vi "打地鼠.vi"() -> ()   [LabVIEW 2022 SP3]
uses:
  <vilib>/Utility/inputDevices.llb/mouseAcquire.vi
panel:
  out "分数":dbl
  out "goal":bool
  out "行":bool
  out "列":bool
  out "axis info":T1 caption="坐标轴信息"
  out "button info":T2 caption="按钮信息"
  in  "取消按钮":bool
  out "数组":bool[][](array[boolean])
  # "左上角135 160\n右上角535 160\n左下角135 540\n右下角535 540\n\n横着：400/5 = 80\n竖着：380/5 = 76\n\n每个格子，是横80竖76"
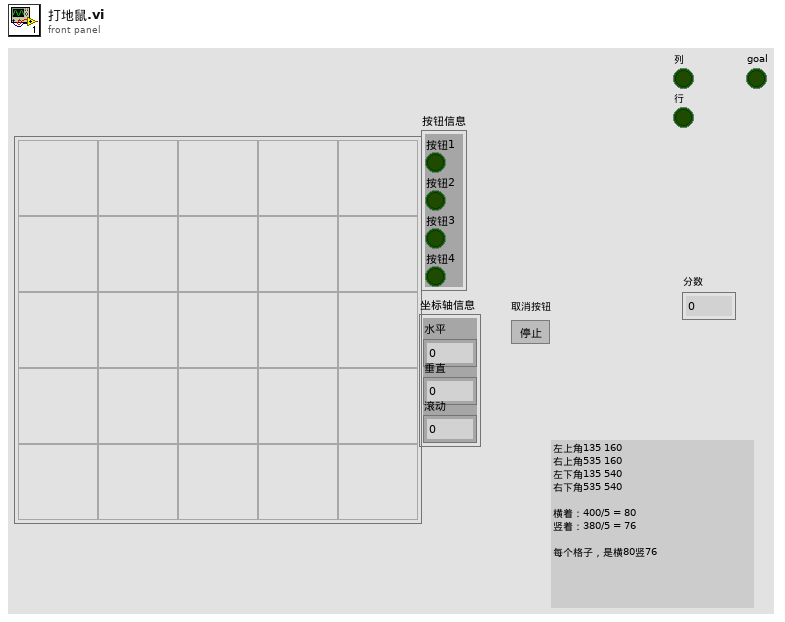
[diagram p1: front panel]
types:
  T1 = cluster{"Horizontal":i32, "Vertical":i32, "Scrolling":i32}
  T2 = cluster{"button 1":bool, "button 2":bool, "button 3":bool, "button 4":bool}
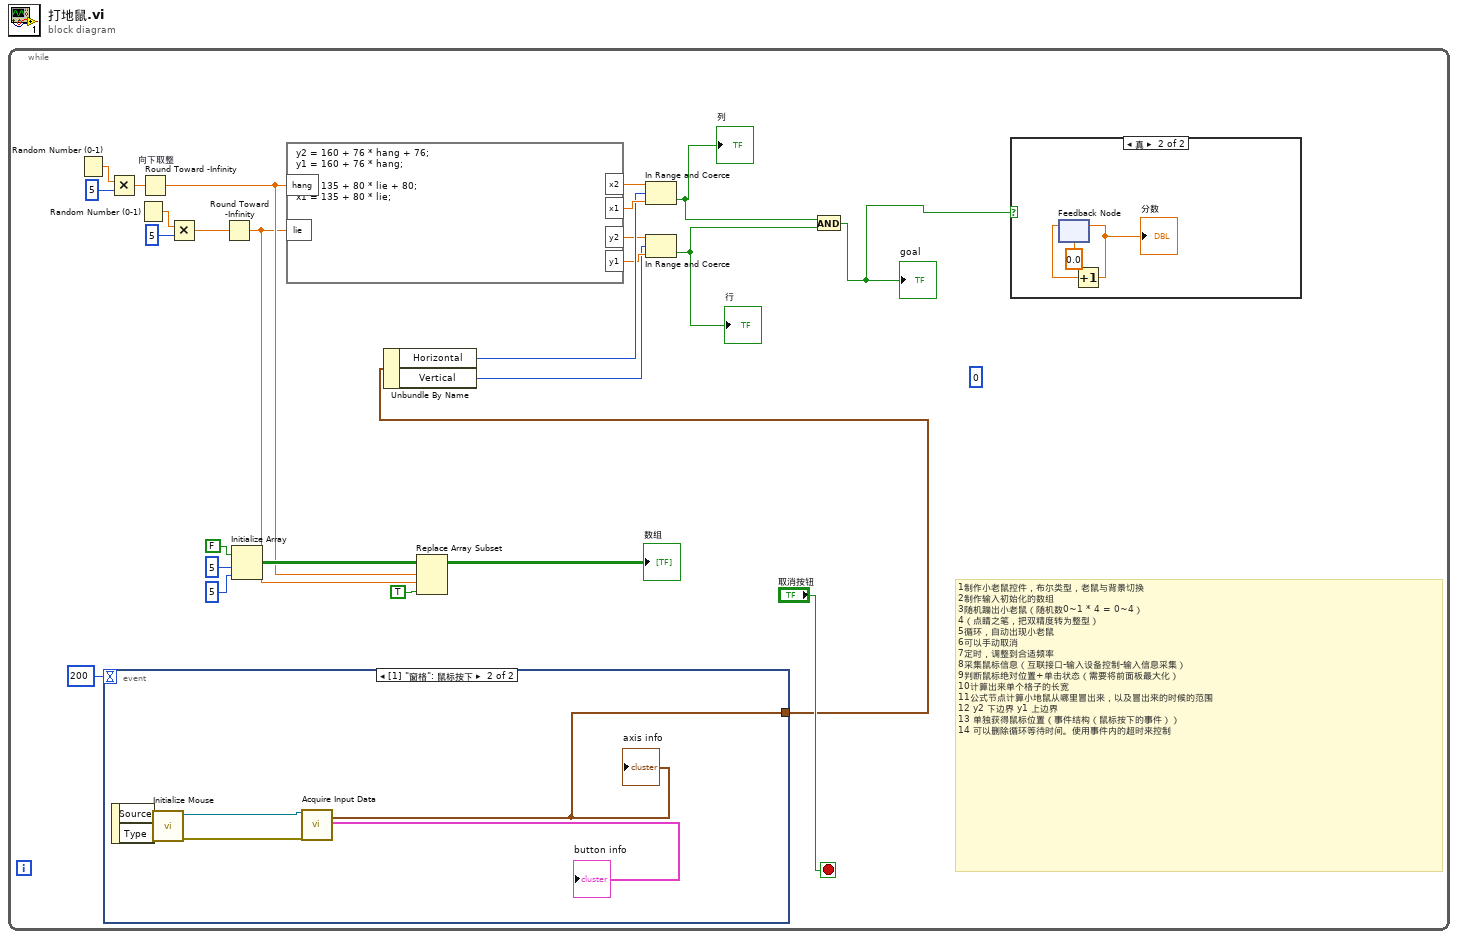
[diagram p0: block diagram]
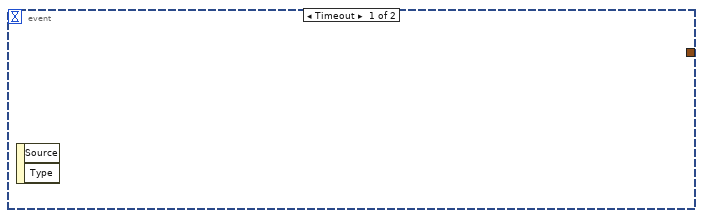
[diagram p3: hidden frame]
diagram:
  n1 = while {
    stop <- "取消按钮" stop-if-true
    (unwired) 0
    # "1制作小老鼠控件，布尔类型，老鼠与背景切换\n2制作输入初始化的数组\n3随机蹦出小老鼠（随机数0~1 * 4 = 0~4）\n4（点睛之笔，把双精度转为整型）\n5循环，自动出现小老鼠\n6可以手动取消\n7定时，调整到合适频率\n8采集鼠标信息（互联接口-输入设备控制-输入信息采集）\n9判断鼠标绝对位置+单击状态（需要将前面板最大化）\n10计算出来单个格子的长宽\n11公式节点计算小地鼠从哪里冒出来，以及冒出来的时候的范围\n12 y2 下边界 y1 上边界\n13 单独获得鼠标位置（事件结构（鼠标按下的事件））\n14 可以删除循环等待时间。使用事件内的超时来控制"
    n2 = Random Number (0-1)() -> (number: 0 to 1=w20:dbl)
    n3 = event shown="[1] \"窗格\": 鼠标按下" {
      selector: _ -> [_ _]
      dyn-events: _ -> [_ _]
      timeout: 200 -> [_ _]
      tunnel: [_ w30] -> w3
      event Timeout {
        n4 = event-data() -> ()  [unwired: 1 in, 2 out]
      }
      event Mouse Down {
        n5 = event-data() -> ()  [unwired: 1 in, 2 out]
        n6 = call <vilib>:"Initialize Mouse.vi"() -> ("error out"=w31:errorcluster, "device ID"=w32:refnum<k1>)  [unwired: 10 in]
        n7 = call-poly <vilib>:"Acquire Input Data.vi"("device ID"=w32, "error in (no error)"=w31) -> ("axis info"=w30:T1, "button info"=→"button info":T2)  [unwired: 14 in, 2 out]
        "axis info" <- w30
      }
    }
    n8 = Multiply(x=w20, y=5) -> (x*y=w16:dbl)
    n9 = Random Number (0-1)() -> (number: 0 to 1=w19:dbl)
    n10 = Round Toward -Infinity "向下取整"(1:w16) -> (0:w7:dbl)
    n11 = Multiply(x=w19, y=5) -> (x*y=w15:dbl)
    n12 = Round Toward -Infinity(1:w15) -> (0:w6:dbl)
    n13 = Initialize Array(FALSE, 5 ("维数大小"), 5 ("维数大小")) -> (w22:bool[][])
    n14 = formula code="y2 = 160 + 76 * hang + 76;\ny1 = 160 + 76 * hang;\n\nx2 = 135 + 80 * lie + 80;\nx1 = 135 + 80 * lie;"("hang"=w7, "lie"=w6) -> ("x2"=w13:dbl, "x1"=w12:dbl, "y2"=w10:dbl, "y1"=w9:dbl)
    n15 = Unbundle By Name(w3) -> ("Horizontal"=w11:i32, "Vertical"=w8:i32)
    n16 = Replace Array Subset(array=w22, new element=TRUE, index (row)=w7, index (col)=w6) -> (→"数组":bool[][])
    n17 = In Range and Coerce(upper limit=w13, x=w11, lower limit=w12) -> (In Range?=w5:bool)  [unwired: 1 out]
    "列" <- w5
    n18 = In Range and Coerce(upper limit=w10, x=w8, lower limit=w9) -> (In Range?=w4:bool)  [unwired: 1 out]
    "行" <- w4
    n19 = And(x=w5, y=w4) -> (x .and. y?=w1:bool)
    "goal" <- w1
    n20 = case shown="真" w1 {
      frame False {
      }
      frame True {
        n21 = feedback #1(0.0) -> (w29:dbl)
        n22 = Increment(x=w29) -> (x+1=w27:dbl)
        "分数" <- w27
        n23 = feedback-in #1(w27) -> ()
      }
    }
  }
